vi "OS_read_four_channels.vi"(0 "VISA resource name":refnum<visa-resource-name>="USB0::0x0699::0x03C6::C010171::INSTR", 1 "Scope Channel 1":T6={"Channel "=1, "Vertical Scale (1.0 V)"=1.0, "Vertical Offset (0.0 V)"=0.0, "Probe Attenuation (1.0)"=1.0, "Coupling (DC)"=1} {"Coupling (DC)" items=["AC", "DC", "GND"]; "Probe Attenuation (1.0)" format="%.1f"; "Vertical Offset (0.0 V)" format="%.3p"; "Vertical Scale (1.0 V)" format="%.3p"; "Channel" items=["Channel 1"=1, "Channel 2"=2, "Channel 3"=3, "Channel 4"=4]}, 2 "Scope Channel 2":T5={"Channel"=2, "Vertical Scale (1.0 V) 2"=1.0, "Vertical Offset (0.0 V) 2"=0.0, "Probe Attenuation (1.0) 2"=1.0, "Coupling (DC) 2"=1} {"Coupling (DC) 2" items=["AC", "DC", "GND"]; "Probe Attenuation (1.0) 2" format="%.1f"; "Vertical Offset (0.0 V) 2" format="%.3p"; "Vertical Scale (1.0 V) 2" format="%.3p"; "Channel" items=["Channel 1"=1, "Channel 2"=2, "Channel 3"=3, "Channel 4"=4]}, 3 "Scope Channel 3":T4={"Channel "=3, "Vertical Scale (1.0 V)"=20.0, "Vertical Offset (0.0 V)"=0.0, "Probe Attenuation (1.0)"=1.0, "Coupling (DC)"=1} {"Coupling (DC)" items=["AC", "DC", "GND"]; "Probe Attenuation (1.0)" format="%.1f"; "Vertical Offset (0.0 V)" format="%.3p"; "Vertical Scale (1.0 V)" format="%.3p"; "Channel" items=["Channel 1"=1, "Channel 2"=2, "Channel 3"=3, "Channel 4"=4]}, 4 "Scope Channel 4":T3={"Channel"=4, "Vertical Scale (1.0 V)"=2.0, "Vertical Offset (0.0 V)"=0.0, "Probe Attenuation (1.0)"=1.0, "Coupling (DC)"=1} {"Coupling (DC)" items=["AC", "DC", "GND"]; "Probe Attenuation (1.0)" format="%.1f"; "Vertical Offset (0.0 V)" format="%.3p"; "Vertical Scale (1.0 V)" format="%.3p"; "Channel" items=["Channel 1"=1, "Channel 2"=2, "Channel 3"=3, "Channel 4"=4]}, 5 "error in (no error)":errorcluster, 6 "Enable Channel 1":bool=TRUE, 7 "Enable Channel 3":bool=TRUE, 8 "Enable Channel 2":bool=TRUE, 9 "Enable Channel 4":bool=TRUE, 10 "Scope Trigger":T2={"Trigger Level (0.0 V)"=0.0, "Trigger Slope (0: Rising)"=0, "Trigger Source (1: Channel 1)"=4, "Trigger Type"=0, "Trigger Coupling"=0, "Trigger Mode"=0} {"Trigger Slope (0: Rising)" items=["Rising", "Falling"]; "Trigger Source (1: Channel 1)" items=["AC Line", "Channel 1", "Channel 2", "Channel 3", "Channel 4"]; "Trigger Type" items=["Edge", "Glitch", "Runt"]; "Trigger Coupling" items=["DC", "HF Rejection", "LF Rejection", "Noise Rejection"]; "Trigger Mode" items=["Auto", "Normal"]}, 11 "Scope Horizontal":T1={"Timebase (4.00 us)"=4e-06, "Delay Time (0.0 s)"=0.0} {"Delay Time (0.0 s)" format="%.2p"; "Timebase (4.00 us)" format="%.2p"}) -> (14 "VISA resource name out":refnum<visa-resource-name>, 16 "Waveform Graph":T7(graph), 19 "error out":errorcluster)   [LabVIEW 2019]
doc: "DESCRIPTION:\nThis VI shows how to configure the oscilloscope for a dual-channel waveform acquisition. It uses edge triggering to trigger the acquisition. \n\nINSTRUCTIONS:\n1. Pass a valid VISA session\n2. Enter a vertical offset, range and coupling for the specified channels.\n3. Enter the probe attenuation for the probe attached to the specified channel inputs.\n4. Enter the delay time and desired time for record you want in the record.\n5. Enter the trigger level and slope for the edge trigger.\n6. Run the VI.\n7. The acquired waveforms will be displayed in the graph."
uses:
  lock-box.llb/Scope Channel 1.ctl
  lock-box.llb/Scope Channel 2.ctl
  lock-box.llb/Scope Channel 3.ctl
  lock-box.llb/Scope Channel 4.ctl
  lock-box.llb/Scope Horizontal.ctl
  <instrlib>/Tektronix TBS 2000 Series/Tektronix TBS 2000 Series.lvlib
panel:
  in  "Acquisition Type":i32(ring) items=["Sample", "Peak Detect", "Average"]
  # "Horizontal Configuration"
  # "Channel A Configuration"
  # "Channel B Configuration"
  # "Triggering (Channel A)"
  # "Channel D Configuration"
  # "Channel C Configuration"
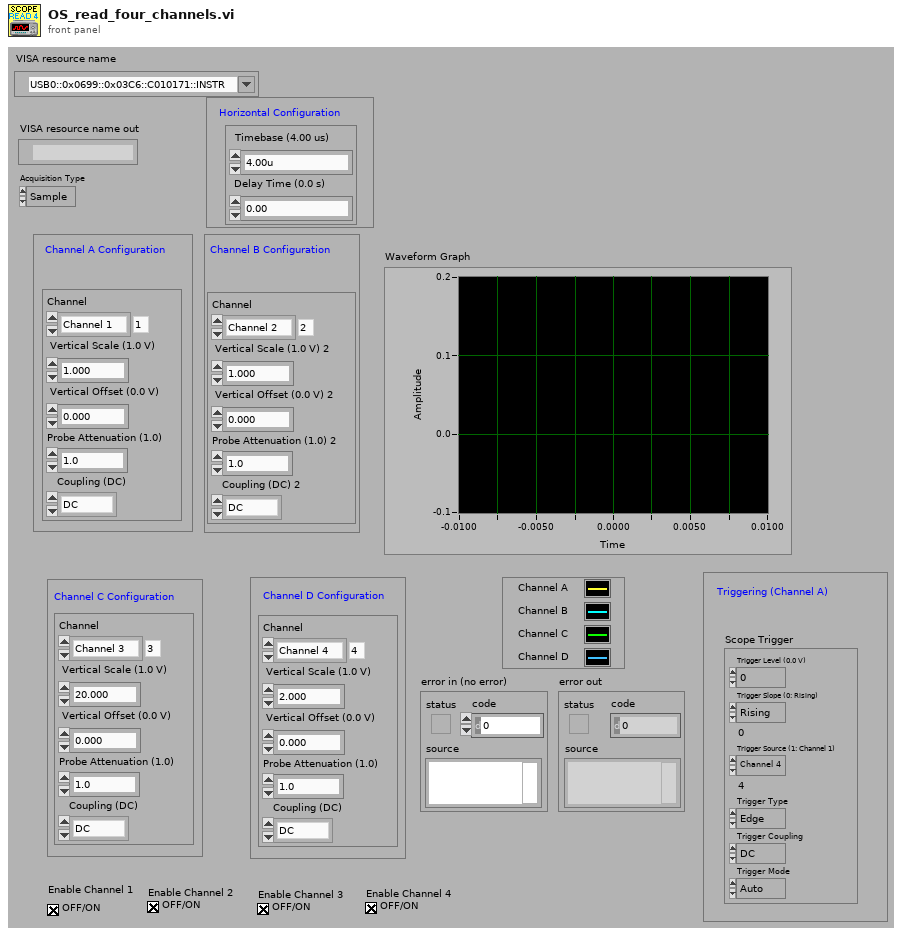
[diagram p1: front panel]
types:
  T1 = typedef "Scope Horizontal.ctl" = cluster{"Timebase (4.00 us)":dbl, "Delay Time (0.0 s)":dbl}
  T2 = cluster{"Trigger Level (0.0 V)":dbl, "Trigger Slope (0: Rising)":i32, "Trigger Source (1: Channel 1)":i32, "Trigger Type":i32, "Trigger Coupling":i32, "Trigger Mode":i32}
  T3 = typedef "Scope Channel 4.ctl" = cluster{"Channel":i32, "Vertical Scale (1.0 V)":dbl, "Vertical Offset (0.0 V)":dbl, "Probe Attenuation (1.0)":dbl, "Coupling (DC)":i32}
  T4 = typedef "Scope Channel 3.ctl" = cluster{"Channel ":i32, "Vertical Scale (1.0 V)":dbl, "Vertical Offset (0.0 V)":dbl, "Probe Attenuation (1.0)":dbl, "Coupling (DC)":i32}
  T5 = typedef "Scope Channel 2.ctl" = cluster{"Channel":i32, "Vertical Scale (1.0 V) 2":dbl, "Vertical Offset (0.0 V) 2":dbl, "Probe Attenuation (1.0) 2":dbl, "Coupling (DC) 2":i32}
  T6 = typedef "Scope Channel 1.ctl" = cluster{"Channel ":i32, "Vertical Scale (1.0 V)":dbl, "Vertical Offset (0.0 V)":dbl, "Probe Attenuation (1.0)":dbl, "Coupling (DC)":i32}
  T7 = cluster{"Initial X":dbl, "X Increment":dbl, "Waveform Array":dbl[]}[]
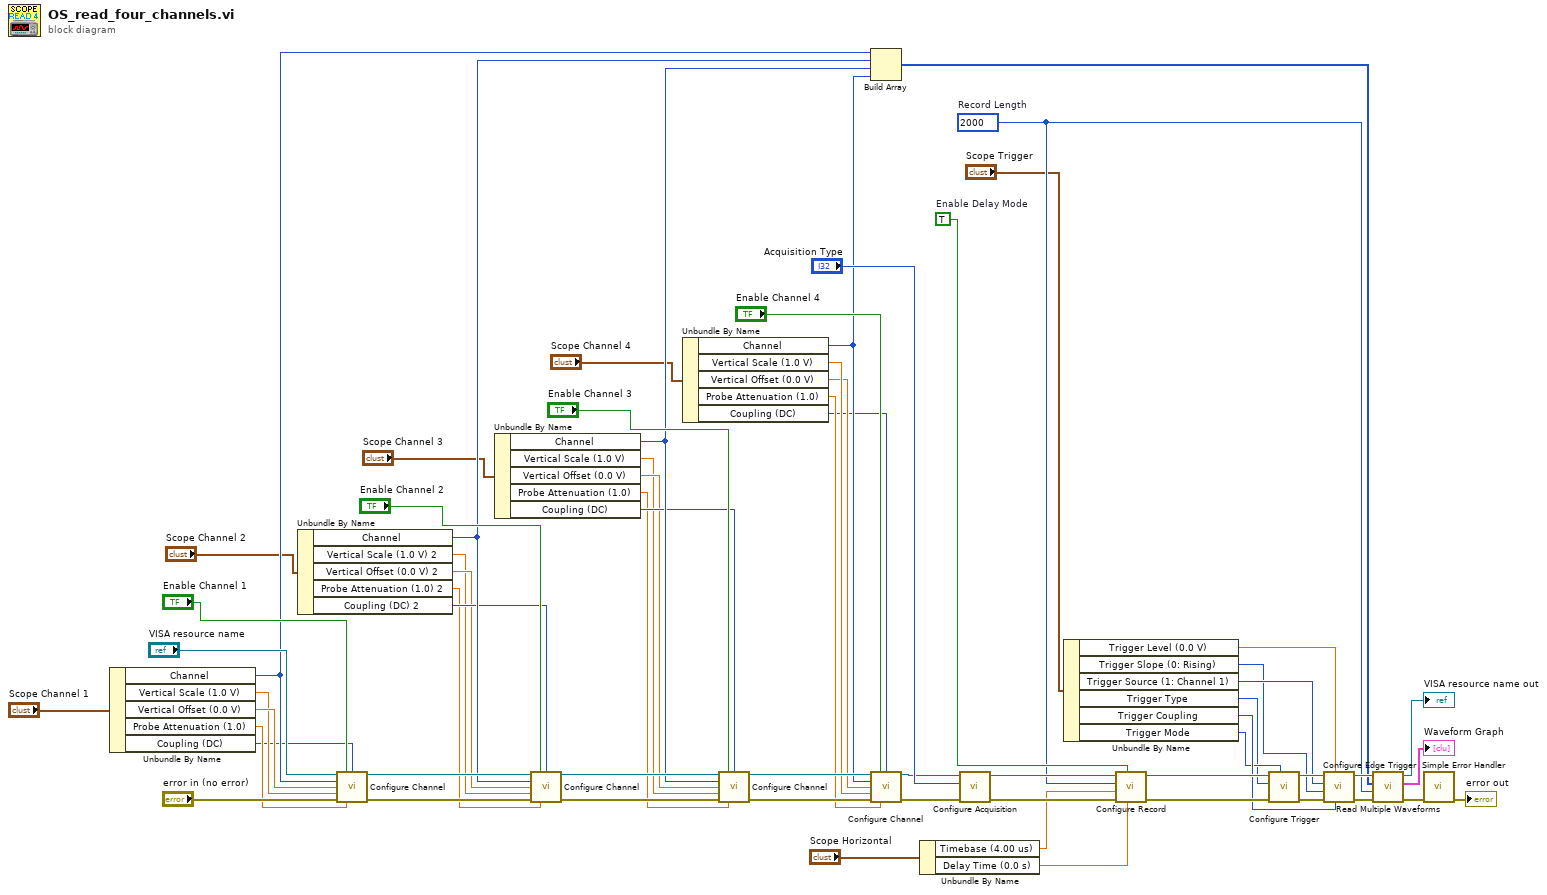
[diagram p0: block diagram]
diagram:
  w49 = TRUE  # Enable Delay Mode
  w48 = 2000 items=["2000"=2000, "20000"=20000, "200000"=200000, "2000000"=2000000, "20000000"=20000000]  # Record Length
  n1 = Unbundle By Name("Scope Channel 1") -> ("Channel"=w33:i32, "Vertical Scale (1.0 V)"=w31:dbl, "Vertical Offset (0.0 V)"=w32:dbl, "Probe Attenuation (1.0)"=w30:dbl, "Coupling (DC)"=w29:i32)
  n2 = Unbundle By Name("Scope Channel 2") -> ("Channel"=w27:i32, "Vertical Scale (1.0 V) 2"=w24:dbl, "Vertical Offset (0.0 V) 2"=w25:dbl, "Probe Attenuation (1.0) 2"=w23:dbl, "Coupling (DC) 2"=w26:i32)
  n3 = call <instrlib>:"Configure Channel.vi"("VISA resource name"="VISA resource name", "Enable Channel (T: Enable)"="Enable Channel 1", "Coupling (1: DC)"=w29, "Channel (1: Channel 1)"=w33, "Vertical Offset (0.0 V)"=w32, "Vertical Scale (1.0 V)"=w31, "error in (no error)"="error in (no error)", "Probe Attenuation (1.0)"=w30) -> ("VISA resource name out"=w63:refnum<visa-resource-name>, "error out"=w64:errorcluster)  [unwired: 6 in]
  n4 = Unbundle By Name("Scope Channel 3") -> ("Channel"=w21:i32, "Vertical Scale (1.0 V)"=w18:dbl, "Vertical Offset (0.0 V)"=w19:dbl, "Probe Attenuation (1.0)"=w17:dbl, "Coupling (DC)"=w20:i32)
  n5 = call <instrlib>:"Configure Channel.vi"("VISA resource name"=w63, "Enable Channel (T: Enable)"="Enable Channel 2", "Coupling (1: DC)"=w26, "Channel (1: Channel 1)"=w27, "Vertical Offset (0.0 V)"=w25, "Vertical Scale (1.0 V)"=w24, "error in (no error)"=w64, "Probe Attenuation (1.0)"=w23) -> ("VISA resource name out"=w40:refnum<visa-resource-name>, "error out"=w39:errorcluster)  [unwired: 6 in]
  n6 = Unbundle By Name("Scope Channel 4") -> ("Channel"=w15:i32, "Vertical Scale (1.0 V)"=w14:dbl, "Vertical Offset (0.0 V)"=w13:dbl, "Probe Attenuation (1.0)"=w12:dbl, "Coupling (DC)"=w11:i32)
  n7 = call <instrlib>:"Configure Channel.vi"("VISA resource name"=w40, "Enable Channel (T: Enable)"="Enable Channel 3", "Coupling (1: DC)"=w20, "Channel (1: Channel 1)"=w21, "Vertical Offset (0.0 V)"=w19, "Vertical Scale (1.0 V)"=w18, "error in (no error)"=w39, "Probe Attenuation (1.0)"=w17) -> ("VISA resource name out"=w38:refnum<visa-resource-name>, "error out"=w37:errorcluster)  [unwired: 6 in]
  n8 = Build Array(w33, w27, w21, w15) -> (w54:i32[])
  n9 = call <instrlib>:"Configure Channel.vi"("VISA resource name"=w38, "Enable Channel (T: Enable)"="Enable Channel 4", "Coupling (1: DC)"=w11, "Channel (1: Channel 1)"=w15, "Vertical Offset (0.0 V)"=w13, "Vertical Scale (1.0 V)"=w14, "error in (no error)"=w37, "Probe Attenuation (1.0)"=w12) -> ("VISA resource name out"=w36:refnum<visa-resource-name>, "error out"=w35:errorcluster)  [unwired: 6 in]
  n10 = Unbundle By Name("Scope Horizontal") -> ("Timebase (4.00 us)"=w2:dbl, "Delay Time (0.0 s)"=w1:dbl)
  n11 = call <instrlib>:"Configure Acquisition.vi"("error in (no error)"=w35, "Acquisition Type (0:Sample)"="Acquisition Type", "VISA resource name"=w36) -> ("error out"=w51:errorcluster, "VISA resource name out"=w50:refnum<visa-resource-name>)  [unwired: 7 in]
  n12 = Unbundle By Name("Scope Trigger") -> ("Trigger Level (0.0 V)"=w6:dbl, "Trigger Slope (0: Rising)"=w7:i32, "Trigger Source (1: Channel 1)"=w9:i32, "Trigger Type"=w4:i32, "Trigger Coupling"=w8:i32, "Trigger Mode"=w5:i32)
  n13 = call <instrlib>:"Configure Record.vi"("Delay Time (0.0 s)"=w1, "Enable Delay Mode (T: Enable)"=w49, "error in (no error)"=w51, "Timebase (4.00 us)"=w2, "Record Length (2000)"=w48, "VISA resource name"=w50) -> ("error out"=w58:errorcluster, "VISA resource name out"=w57:refnum<visa-resource-name>)  [unwired: 4 in]
  n14 = call <instrlib>:"Configure Trigger.vi"("Trigger Mode (0: Auto)"=w5, "error in (no error)"=w58, "Trigger Type (0: Edge)"=w4, "VISA resource name"=w57) -> ("error out"=w61:errorcluster, "VISA resource name out"=w62:refnum<visa-resource-name>)  [unwired: 6 in]
  n15 = call <instrlib>:"Configure Edge Trigger.vi"("Trigger Coupling (0: DC)"=w8, "Trigger Level (0.0 V)"=w6, "error in (no error)"=w61, "Trigger Slope (0: Rising)"=w7, "Trigger Source (1: Channel 1)"=w9, "VISA resource name"=w62) -> ("error out"=w56:errorcluster, "VISA resource name out"=w55:refnum<visa-resource-name>)  [unwired: 4 in]
  n16 = call <instrlib>:"Read Multiple Waveforms.vi"("error in (no error)"=w56, "Waveform End (2000)"=w48, "Sources"=w54, "VISA resource name"=w55) -> ("error out"=w44:errorcluster, "Waveform Graph"=→"Waveform Graph":T7, "VISA resource name out"=→"VISA resource name out":refnum<visa-resource-name>)  [unwired: 5 in]
  n17 = call <vilib>:"Simple Error Handler.vi"("error in (no error)"=w44) -> ("error out"=→"error out":errorcluster)  [unwired: 4 in, 4 out]
